vi "solar Rendezvous.vi"(8 "error in (no error)":errorcluster, 9 "Timeout (10000ms)":u32=10000, 11 "solar in":refnum<class "solar.lvclass">) -> (0 "error out":errorcluster, 1 "Timed Out?":bool, 2 "Shared":variant, 3 "solar out":refnum<class "solar.lvclass">)   [LabVIEW 2018, in "solar.lvclass"]
doc: "Handle target rendezvous."
uses:
  solar.lvclass
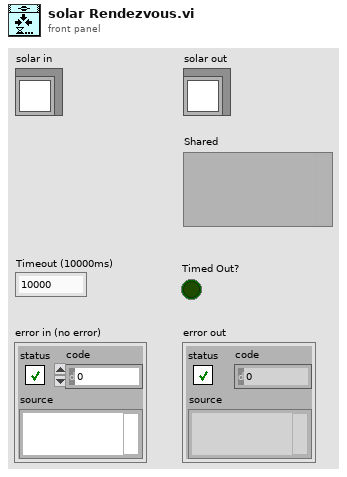
[diagram p1: front panel]
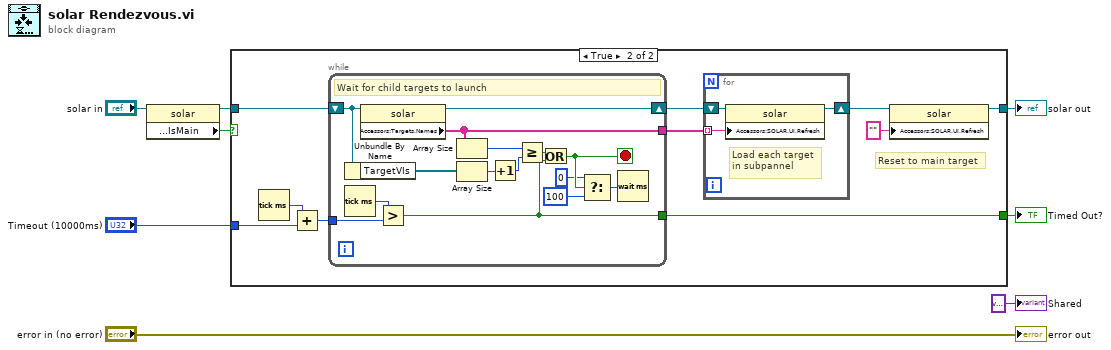
[diagram p0: block diagram]
diagram:
  n1 = property class="solar"(reference="solar in") -> (reference out=w4:refnum<class "solar.lvclass">, "Accessors:Main.IsMain"=w1:bool)  [unwired: 1 in, 1 out]
  n2 = case shown="True" w1 {
    tunnel: [w9 w19] -> w5
    tunnel: w4 -> [w9 w16]
    tunnel: "Timeout (10000ms)" -> [_ w14]
    tunnel: [_ w12] -> w2
    frame False {
    }
    frame True {
      # "Reset to main target"
      n3 = Tick Count (ms)() -> (millisecond timer value=w15:u32)
      n4 = Add(x=w15, y=w14) -> (x+y=w13:u32)
      n5 = while {
        shift-right: [w35] -> w17
        shift-left: w16 -> [w31]
        tunnel: w13 -> [w29]
        tunnel: [w28] -> w12
        tunnel: [w23] -> w10
        stop <- w27 stop-if-true
        # "Wait for child targets to launch"
        n6 = Unbundle By Name(w31) -> ("TargetVIs"=w37:refnum<vi>[])
        n7 = Tick Count (ms)() -> (millisecond timer value=w30:u32)
        n8 = property class="solar"(reference=w31) -> (reference out=w35:refnum<class "solar.lvclass">, "Accessors:Targets.Names"=w23:string[])  [unwired: 1 in, 1 out]
        n9 = Greater?(x=w30, y=w29) -> (0:w28:bool)
        n10 = Array Size(array=w23) -> (size(s)=w33:i32)
        n11 = Array Size(array=w37) -> (size(s)=w36:i32)
        n12 = Increment(x=w36) -> (x+1=w34:i32)
        n13 = Greater Or Equal?(x=w33, y=w34) -> (x >= y?=w32:bool)
        n14 = Or(x=w32, y=w28) -> (x .or. y?=w27:bool)
        n15 = Select(t=u32 0 ("milliseconds to wait"), s=w27, f=u32 100 ("milliseconds to wait")) -> (s? t:f=w24:u32)
        n16 = Wait (ms)(milliseconds to wait=w24) -> ()  [unwired: 1 out]
      }
      n17 = for {
        shift-right: [w21] -> w11
        shift-left: w17 -> [w22]
        tunnel: w10 -> [w20] mode=indexing
        # "Load each target\nin subpannel"
        n18 = property class="solar"(reference=w22, "Accessors:SOLAR.UI.Refresh"=w20) -> (reference out=w21:refnum<class "solar.lvclass">)  [unwired: 1 in, 1 out]
      }
      n19 = property class="solar"(reference=w11, "Accessors:SOLAR.UI.Refresh"="" ("SOLAR:UI:Refresh")) -> (reference out=w19:refnum<class "solar.lvclass">)  [unwired: 1 in, 1 out]
    }
  }
  "solar out" <- w5
  "Timed Out?" <- w2
  "error out" <- "error in (no error)"
  "Shared" <- variant ("Shared")
